vi "ArgoBot_Main.vi"() -> ()   [LabVIEW 2016]
uses:
  ArgoBotLib.lvlib
panel:
  in  "Setup":T1={"Analog 1 Config"=1, "Analog 2 Config"=1, "Analog 3 Config"=1, "GPIO 1 Config"=0, "GPIO 2 Config"=0, "GPIO 3 Config"=0, "Drive Config"=0, "Motor Mode"=0, "Battery_Config"=1, "LED Config"=0} {"Drive Config" items=["Off", "On"]; "Motor Mode" items=["Coast", "Brake"]; "Battery_Config" items=["Off", "On"]; "LED Config" items=["Blink", "Write"]; "Analog 3 Config" items=["Read", "Off"]; "Analog 1 Config" items=["Read", "Off"]; "Analog 2 Config" items=["Read", "Off"]; "GPIO 1 Config" items=["Off", "Read", "Write", "PWM ", "Servo"]; "GPIO 2 Config" items=["Off", "Read", "Write", "PWM ", "Servo"]; "GPIO 3 Config" items=["Off", "Read", "Write", "PWM ", "Servo"]}
  out "Read_Value":T2 {"Voltage" scale=0.0..6.5; "Analog 1" format="%#_2g"; "Analog 2" format="%#_2g"; "Analog 3" format="%#_2g"; "Loop Rate (Hz)" scale=0.0..50.0}
  in  "stop":bool
  # "http://playingwithfusion.com"
  # "ArgoBot"
  # "http://playingwithfusion.com"
  # "Instructions\n1.\tConnect the provided router (USB and Ethernet cable)\n2. Wait for the green light to turn solid\n2.\tTurn on ArgoBot and wait 10 seconds\n3.\tStart Labview by clicking the Run Arrow in the upper left hand corner"
  # "Battery Voltage"
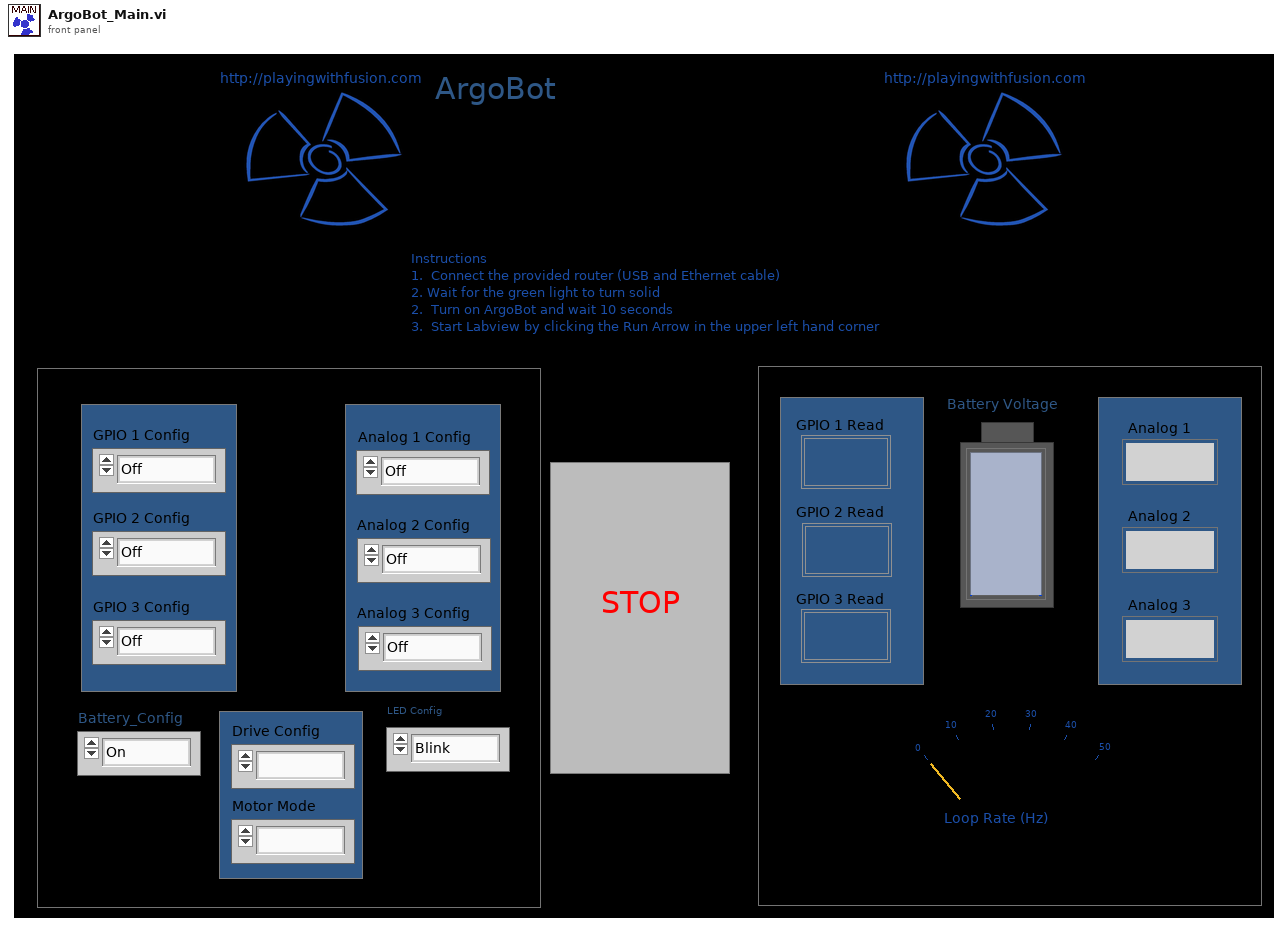
[diagram p1: front panel]
types:
  T1 = cluster{"Analog 1 Config":u16, "Analog 2 Config":u16, "Analog 3 Config":u16, "GPIO 1 Config":u16, "GPIO 2 Config":u16, "GPIO 3 Config":u16, "Drive Config":u16, "Motor Mode":u16, "Battery_Config":u16, "LED Config":u16}
  T2 = cluster{"Analog 1":dbl, "Analog 2":dbl, "Analog 3":dbl, "Voltage":dbl, "GPIO 1 Read":bool, "GPIO 2 Read":bool, "GPIO 3 Read":bool, "Loop Rate (Hz)":u32}
  T3 = typedef "LMH-LINX.lvlib/LINX Ref.ctl" = cluster{"IO":T4, "Interface":T5, "LINX Device Config":T6}
  T4 = typedef "LMH-LINX.lvlib/Platform.ctl" = enum16{"Remote", "Local"}
  T5 = typedef "LMH-LINX.lvlib/Interface.ctl" = enum16{"Serial", "TCP"}
  T6 = typedef "LMH-LINX.lvlib/Device.lvlib/LINX Device Config.ctl" = cluster{"Interface":T5, "COM Port":refnum<visa-resource-name>, "TCP Configuration":T7, "Device Family":u8, "Device ID":u8, "Device Name":string, "TCP Ref":refnum<k5>, "Channels":T8}
  T7 = typedef "LMH-LINX.lvlib/Device.lvlib/TCP Config.ctl" = cluster{"IP Address":string, "Port":u16}
  T8 = typedef "LMH-LINX.lvlib/Channels.ctl" = cluster{"DI":u8[], "DO":u8[], "AI":u8[], "AO":u8[], "PWM":u8[], "QE":u8[], "UART":u8[], "I2C 2":u8[], "SPI":u8[], "CAN":u8[], "Servo":u8[], "AI Ref (V)":dbl, "AI Resolution (Bits)":u8, "AO Ref (V)":dbl, "AO Resolution (Bits)":u8}
  T9 = cluster{"Joystick error out":errorcluster, "Linx":cluster{"LINX Ref":T3, "Error Out":errorcluster}, "Setup":cluster{"Analog 1 Config":u16, "Analog 2 Config":u16, "Analog 3 Config":u16, "GPIO 1 Config":u16, "GPIO 2 Config":u16, "GPIO 3 Config":u16, "Drive Config":u16, "Motor Mode":u16, "Battery_Config":u16, "LED Config":u16}}
  T10 = cluster{"Joystick Read":cluster{"Joystick":cluster{"A":bool, "B":bool, "X":bool, " Y":bool, "Left_Trigger":dbl, "Right_Trigger ":dbl, "LB":bool, " RB":bool, "Left_Thumb_Button":bool, "Right_Thumb_Button":bool, "Stop_Back":bool, "Start":bool, "X_Axis_Left":dbl, "Y_Axis_Left":dbl, "X_Axis_Right":dbl, "Y_Axis_Right":dbl}, "Joystick error out":errorcluster, "Refnum out":refnum<k1>}, "Read Config":cluster{"Read_Config":i32[], "Error Out":errorcluster, "LINX Resource 2":T3}, "Read_Value":cluster{"Analog 1":dbl, "Analog 2":dbl, "Analog 3":dbl, "Voltage":dbl, "GPIO 1 Read":bool, "GPIO 2 Read":bool, "GPIO 3 Read":bool, "Loop Rate (Hz)":u32}, "Joystick error out":errorcluster, "Linx":cluster{"LINX Ref":T3, "Error Out":errorcluster}, "Setup":cluster{"Analog 1 Config":u16, "Analog 2 Config":u16, "Analog 3 Config":u16, "GPIO 1 Config":u16, "GPIO 2 Config":u16, "GPIO 3 Config":u16, "Drive Config":u16, "Motor Mode":u16, "Battery_Config":u16, "LED Config":u16}}
  T11 = cluster{"Output Confic":cluster{"Error Out":errorcluster, "LINX Resource":T3}, "Joystick Read":cluster{"Joystick":cluster{"A":bool, "B":bool, "X":bool, " Y":bool, "Left_Trigger":dbl, "Right_Trigger ":dbl, "LB":bool, " RB":bool, "Left_Thumb_Button":bool, "Right_Thumb_Button":bool, "Stop_Back":bool, "Start":bool, "X_Axis_Left":dbl, "Y_Axis_Left":dbl, "X_Axis_Right":dbl, "Y_Axis_Right":dbl}, "Joystick error out":errorcluster, "Refnum out":refnum<k1>}, "Read Config":cluster{"Read_Config":i32[], "Error Out":errorcluster, "LINX Resource 2":T3}, "Read_Value":cluster{"Analog 1":dbl, "Analog 2":dbl, "Analog 3":dbl, "Voltage":dbl, "GPIO 1 Read":bool, "GPIO 2 Read":bool, "GPIO 3 Read":bool, "Loop Rate (Hz)":u32}, "Joystick error out":errorcluster, "Linx":cluster{"LINX Ref":T3, "Error Out":errorcluster}, "Setup":cluster{"Analog 1 Config":u16, "Analog 2 Config":u16, "Analog 3 Config":u16, "GPIO 1 Config":u16, "GPIO 2 Config":u16, "GPIO 3 Config":u16, "Drive Config":u16, "Motor Mode":u16, "Battery_Config":u16, "LED Config":u16}}
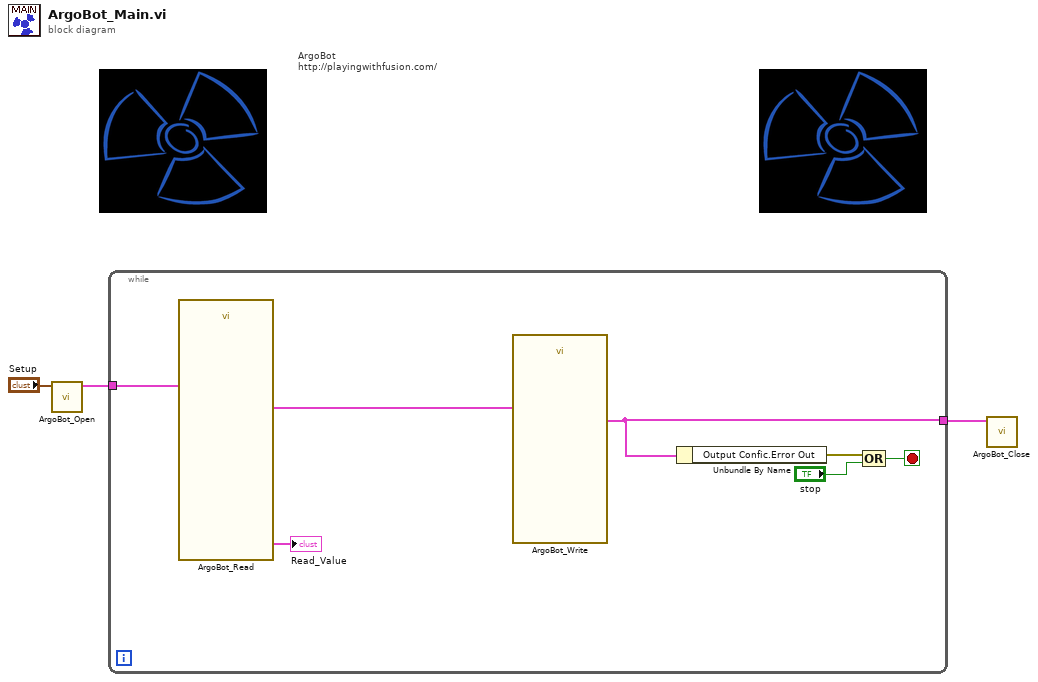
[diagram p0: block diagram]
diagram:
  # "ArgoBot\nhttp://playingwithfusion.com/"
  n1 = call "ArgoBot_Open.vi"("Setup"="Setup") -> ("Open_Cluster"=w3:T9)  [unwired: 10 in]
  n2 = while {
    tunnel: w3 -> [w7]
    tunnel: [w5] -> w2
    stop <- w9 stop-if-true
    n3 = call "ArgoBot_Read.vi"("Open_Cluster"=w7) -> ("Read_Value"=→"Read_Value":T2, "Read_Cluster"=w4:T10)  [unwired: 2 in, 7 out]
    n4 = call "ArgoBot_Write.vi"("Read_Cluster"=w4) -> ("Write Cluster"=w5:T11)  [unwired: 10 in]
    n5 = Unbundle By Name(w5) -> ("Output Confic.Error Out"=w10:errorcluster)
    n6 = Compound Arithmetic op=OR(w10, "stop") -> (w9:bool)
  }
  n7 = call "ArgoBot_Close.vi"("Write_Cluster"=w2) -> ()  [unwired: 11 in]
